vi "Send Debug Info to DETT.vi"(6 "f":string, 8 "Heart Rate Timer":i32, 9 "Last Slope":dbl, 10 "Slope":dbl, 11 "Pulse":bool) -> ()   [LabVIEW 2017]
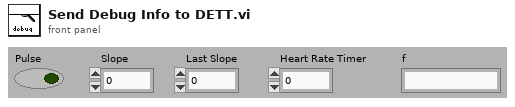
[diagram p1: front panel]
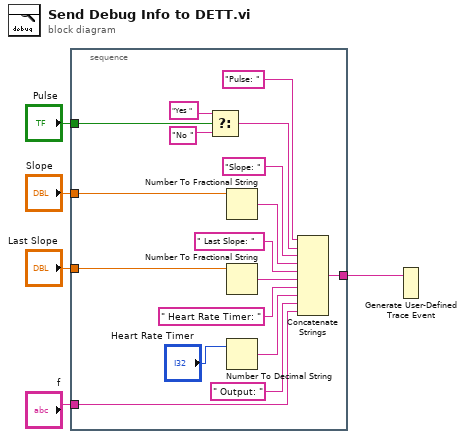
[diagram p0: block diagram]
diagram:
  n1 = stacked-sequence {
    tunnel: "f" -> [w22]
    tunnel: "Last Slope" -> [w16]
    tunnel: "Slope" -> [w13]
    tunnel: "Pulse" -> [w8]
    tunnel: [w6] -> w1
    frame #0 {
      n2 = Select(t="Yes " ("string"), s=w8, f="No " ("string")) -> (s? t:f=w11:string)
      n3 = Number To Fractional String(number=w13) -> (F-format string=w14:string)  [unwired: 3 in]
      n4 = Number To Fractional String(number=w16) -> (F-format string=w17:string)  [unwired: 3 in]
      n5 = Number To Decimal String(number="Heart Rate Timer") -> (decimal integer string=w20:string)  [unwired: 1 in]
      n6 = Concatenate Strings("Pulse: " ("string"), w11, "Slope: " ("string"), w14, " Last Slope: " ("string"), w17, " Heart Rate Timer: " ("string"), w20, " Output: " ("string"), w22) -> (w6:string)
    }
  }
  n7 = Generate User-Defined Trace Event(2:w1) -> ()  [unwired: 1 in]
